vi "comm termination.vi"(8 "error in (no error)":errorcluster, 9 "termination characters":string, 10 "Termination Character Enable":bool, 11 "Comm Handle":u64) -> (0 "error out":errorcluster, 3 "dup Comm Handle":u64)   [LabVIEW 2021, in "lvserial.lvlib"]
doc: "Configures the termiation characters for the serial port."
uses:
  lvserial.lvlib
  lvserial.dll
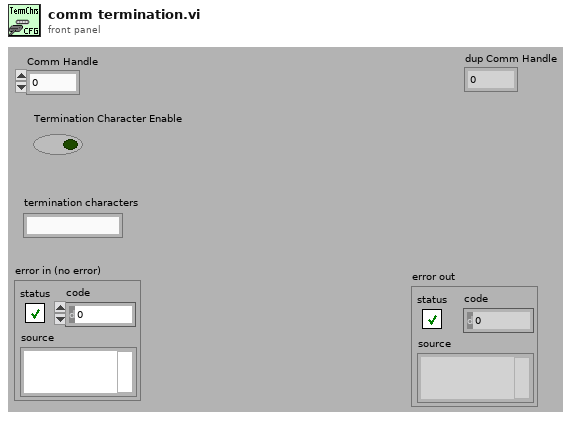
[diagram p1: front panel]
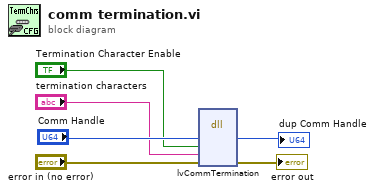
[diagram p0: block diagram]
diagram:
  n1 = dll-call lib="lvserial.dll" fn="lvCommTermination"("hComm"="Comm Handle", "lfTermCharEnable"="Termination Character Enable", "pcTermCharacter"="termination characters", "error"="error in (no error)") -> ("hComm"=→"dup Comm Handle":u64, "error"=→"error out":errorcluster)  [unwired: 5 in, 3 out]
